vi "Poll Front Panel Change.vi"(0 "Display State In":T1, 5 "First call?":bool, 9 "Container State":T2, 11 "error in (no error)":errorcluster) -> (4 "Display State Out":T1, 15 "error out":errorcluster)   [LabVIEW 2015, in "Dynamic Device List.xctl"]
uses:
  Dynamic Device List.xctl
  <vilib>/_xctls/Container State.ctl
  Dynamic FP container.llb/Dynamic FP State.ctl
  Device/Device.lvclass
  <vilib>/_xctls/XControlSupport.lvlib
panel:
  # "Add Controls & Indicators that form the parameters of the method here. Hook them to the connector pane. Do not delete the controls & indicators that are already hooked to the connector pane.\n \nTo setup the parameters  for this method, right click on this item in the Project Tree & select \"Configure Method...\"."
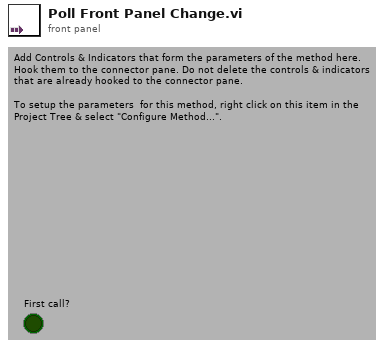
[diagram p1: front panel]
types:
  T1 = typedef "Dynamic Device List.xctl/Dynamic FP State.ctl" = cluster{"Complete device list":refnum<class "Device.lvclass">[], "Boolean test":bool, "Selected devices":u16[]}
  T2 = typedef "XControlSupport.lvlib/Container State.ctl" = cluster{"Indicator?":bool, "Run Mode?":bool, " Refnum":refnum<vi>}
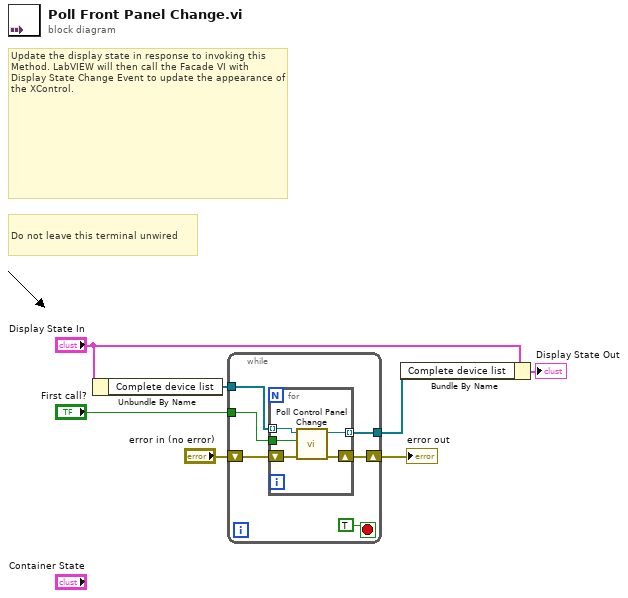
[diagram p0: block diagram]
diagram:
  # "Do not leave this terminal unwired"
  # "Update the display state in response to invoking this Method. LabVIEW will then call the Facade VI with Display State Change Event to update the appearance of the XControl."
  n1 = Unbundle By Name("Display State In") -> ("Complete device list"=w7:refnum<class "Device.lvclass">[])
  n2 = while {
    tunnel: w7 -> [w13]
    shift-right: [w9] -> w5
    shift-left: "error in (no error)" -> [w11]
    tunnel: "First call?" -> [w10]
    tunnel: [w8] -> w2
    stop <- TRUE stop-if-true
    n3 = for {
      tunnel: w13 -> [w15] mode=indexing
      shift-right: [w17] -> w9
      shift-left: w11 -> [w18]
      tunnel: w10 -> [w14]
      tunnel: [w16] -> w8 mode=indexing
      n4 = call "Poll Control Panel Change.vi"("error in (no error)"=w18, "First call?"=w14, "Device"=w15) -> ("error out"=w17:errorcluster, "Device out"=w16:refnum<class "Device.lvclass">)  [unwired: 7 in]
    }
  }
  "error out" <- w5
  n5 = Bundle By Name(cluster="Display State In", "Complete device list"=w2) -> (→"Display State Out":T1)
